vi "Format Control Table.vi"(5 "Msg Chain in":string, 7 "Controls Opt":T4, 8 "error in (no error)":errorcluster {"code" format="Error %.0f"}, 10 "Controls":T1[](array[typedef]), 11 "VIDoc Printer - Confluence In":refnum<class "VIDoc Printer - Confluence.lvclass">) -> (0 "error out":errorcluster {"code" format="Error %.0f"}, 2 "Table":string, 3 "VIDoc Printer - Confluence Out":refnum<class "VIDoc Printer - Confluence.lvclass">)   [LabVIEW 2023, in "VIDoc Printer - Confluence.lvlib" / "VIDoc Printer - Confluence.lvclass"]
uses:
  VIDoc Printer - Confluence.lvclass
  C:/projects/DMC/GitHub/DMC CLI VIDoc/Source/Documentation Generation/Printers/Printer/VIDoc Printer.lvclass
  Settings/Printer Settings/Detail Level Enum.ctl
  Parsing/TypeDefs/Controls Info Cluster.ctl
  <vilib>/picture/picture.llb/imagedata.ctl
  <vilib>/Utility/miscctls.llb/LVKeyTypeDef.ctl
  VIDoc Printer - Confluence.lvclass/VIDoc Printer - Confluence.ctl
  Accessors/Get Control Column Ordering - Full.vi
  Accessors/Get Control Column Ordering - Minimal.vi
  Accessors/Get Control Column Ordering - Standard.vi
  Accessors/Get Sortable Tables.vi
  Confluence Formatting/Confluence Formatting.lvlib
  Printer/VIDoc Printer.lvclass
  UI Interaction/UI Interaction.lvclass
  Parsing/VIDoc Parsing.lvlib
  Settings/Printer Settings/Printer Settings.lvclass
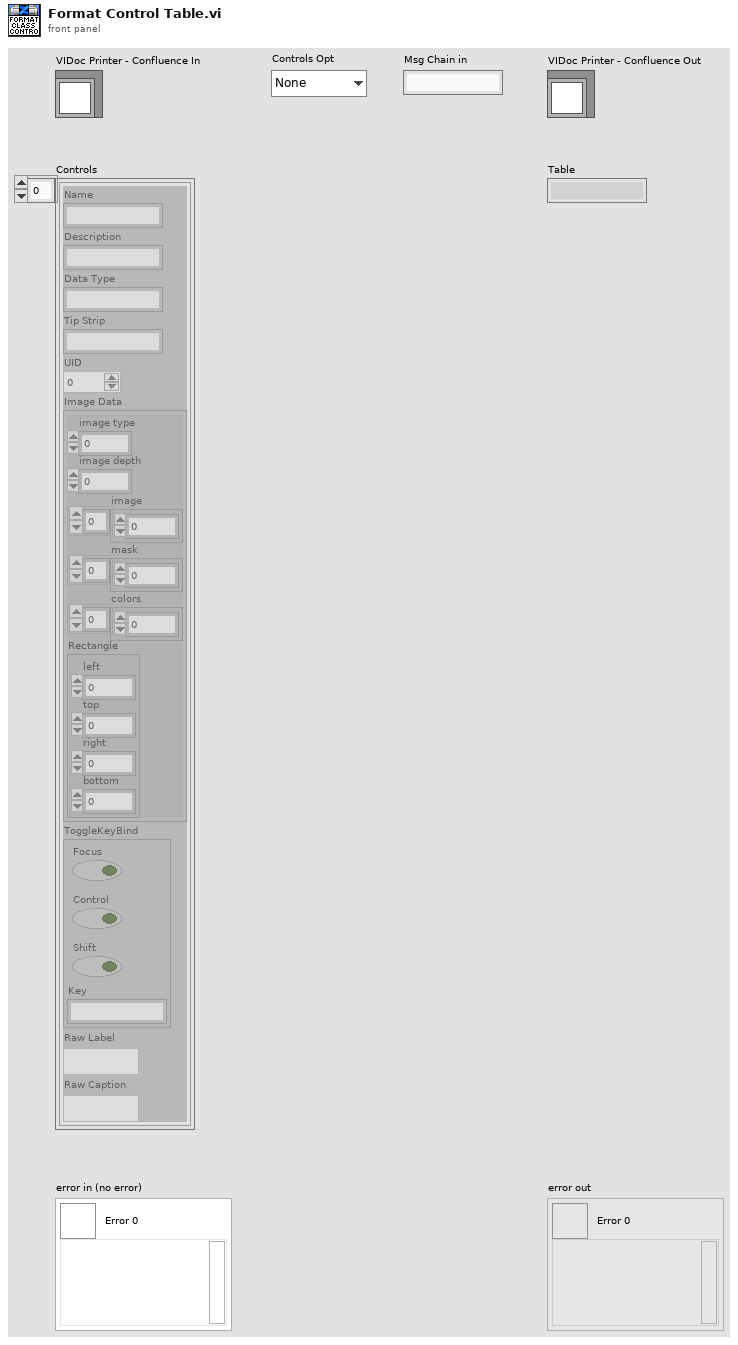
[diagram p1: front panel]
types:
  T1 = typedef "VIDoc Parsing.lvlib/Controls Info Cluster.ctl" = cluster{"Name":string, "Description":string, "Data Type":string, "Tip Strip":string, "UID":i32, "Image Data":T2, "ToggleKeyBind":T3, "Raw Label":string, "Raw Caption":string}
  T2 = typedef "imagedata.ctl" = cluster{"image type":i32, "image depth":i32, "image":u8[], "mask":u8[], "colors":u32[], "Rectangle":cluster{"left":i16, "top":i16, "right":i16, "bottom":i16}}
  T3 = typedef "LVKeyTypeDef.ctl" = cluster{"Focus":bool, "Control":bool, "Shift":bool, "Key":string}
  T4 = typedef "VIDoc Printer.lvlib/Printer Settings.lvclass/Detail Level Enum.ctl" = enum16{"None", "Minimal", "Standard", "Full"}
  T5 = typedef "VIDoc Printer - Confluence.lvlib/VIDoc Settings - Confluence.lvclass/Control Info Column.ctl" = enum16{"Image", "Name", "Description", "Caption", "Tip Strip", "Data Type", "Key Toggle"}
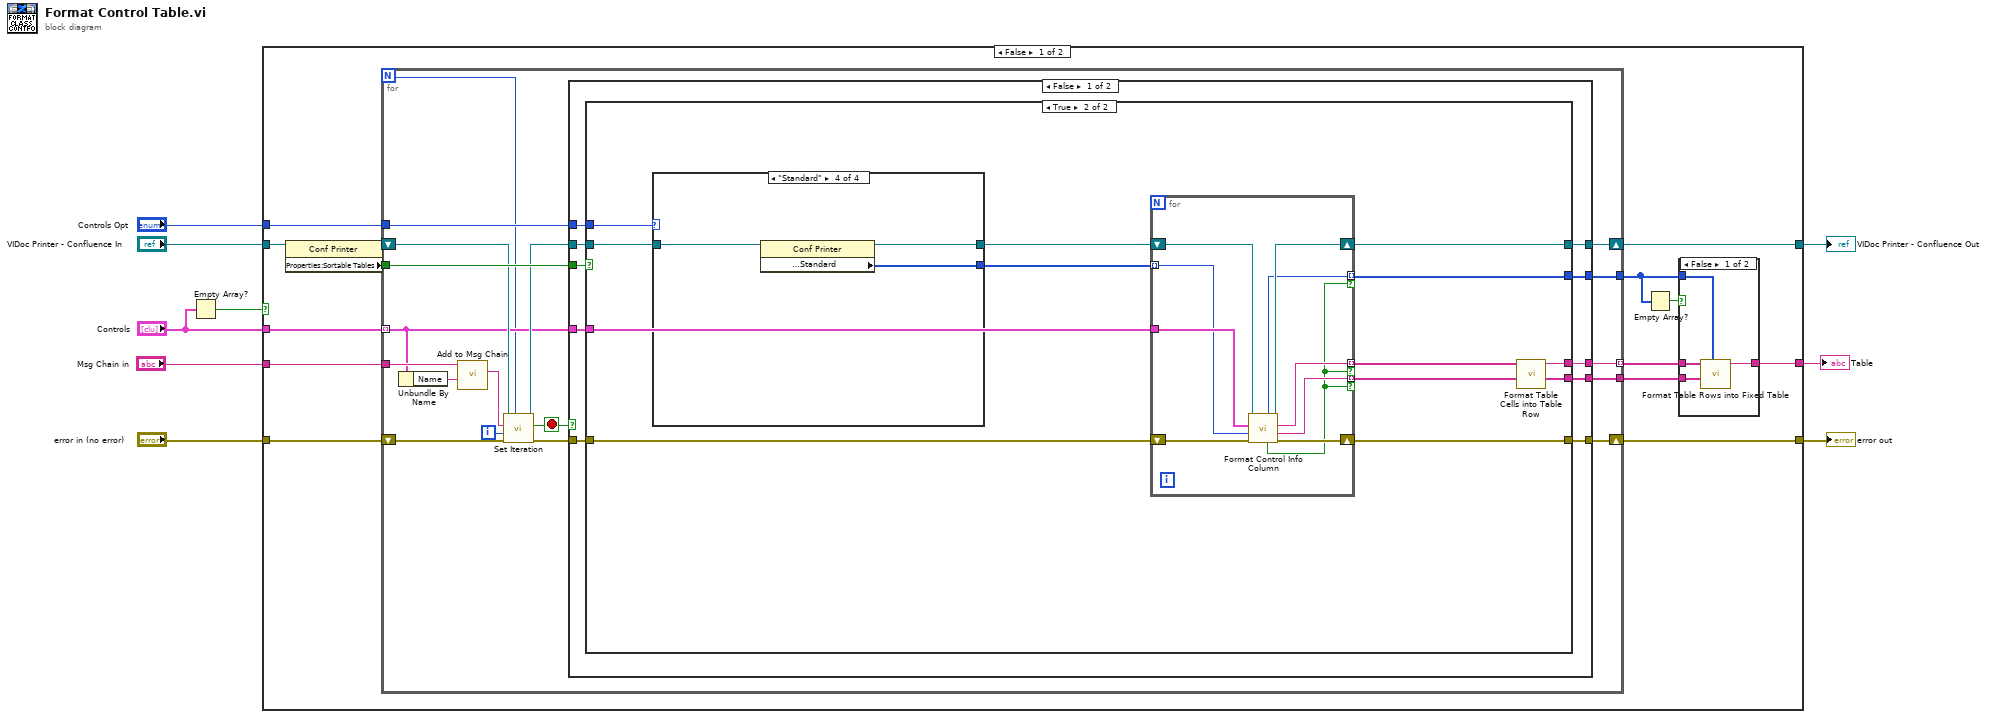
[diagram p0: block diagram]
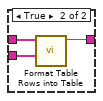
[diagram p2: hidden frame]
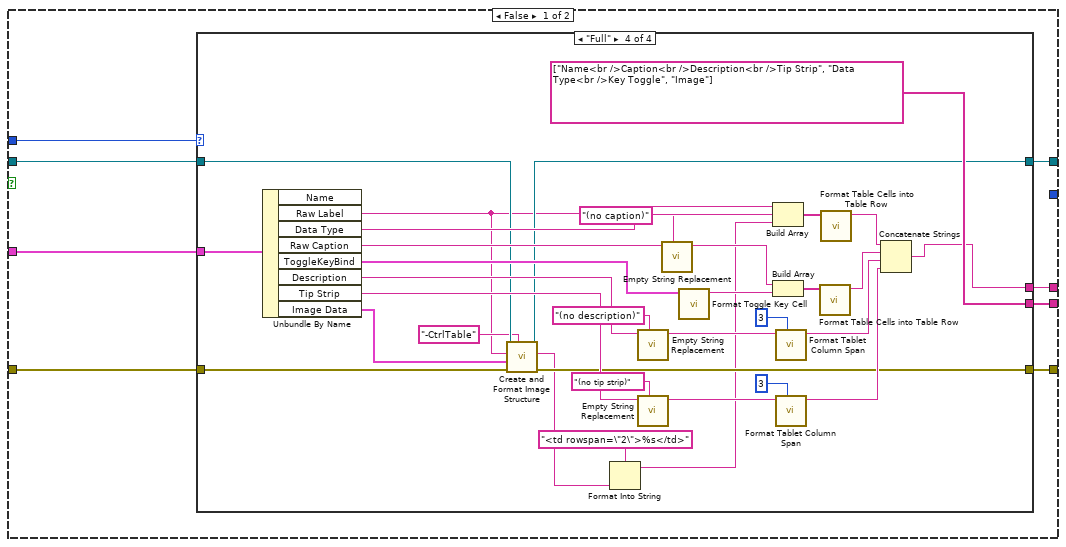
[diagram p3: hidden frame]
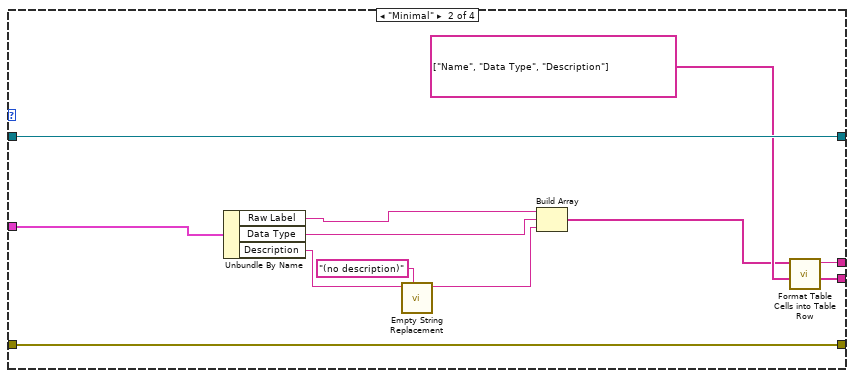
[diagram p5: hidden frame]
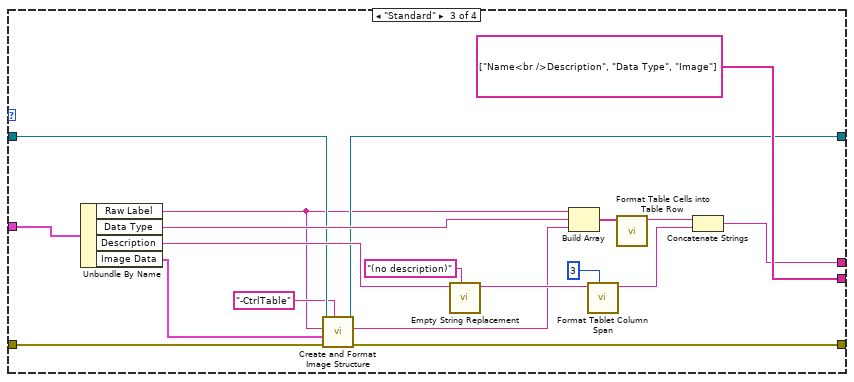
[diagram p6: hidden frame]
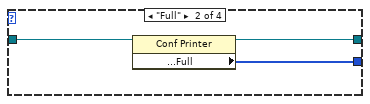
[diagram p8: hidden frame]
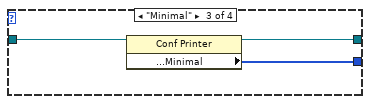
[diagram p9: hidden frame]
diagram:
  n1 = Empty Array?(array="Controls") -> (empty?=w3:bool)
  n2 = case shown="False" w3 {
    tunnel: "Controls Opt" -> [w23 _]
    tunnel: [w22 w166] -> w8
    tunnel: "error in (no error)" -> [w17 w166]
    tunnel: [w21 w167] -> w6
    tunnel: "VIDoc Printer - Confluence In" -> [w20 w167]
    tunnel: [w13 _] -> w4
    tunnel: "Controls" -> [w19 _]
    tunnel: "Msg Chain in" -> [w15 _]
    frame False {
      n3 = property class="Conf Printer"(reference=w20) -> (reference out=w16:refnum<class "VIDoc Printer - Confluence.lvclass">, "Properties:Sortable Tables"=w18:bool)  [unwired: 1 in, 1 out]
      n4 = for {
        N -> [w36]
        tunnel: w23 -> [w48]
        tunnel: w19 -> [w37] mode=indexing
        tunnel: w18 -> [w45]
        tunnel: w15 -> [w38]
        shift-right: [w47] -> w22
        shift-left: w17 -> [w42]
        shift-right: [w46] -> w21
        shift-left: w16 -> [w40]
        tunnel: [w33] -> w12 mode=indexing
        tunnel: [w32] -> w11
        tunnel: [w31] -> w10
        i -> [w35]
        stop <- w34 stop-if-true
        n5 = Unbundle By Name(w37) -> ("Name"=w44:string)
        n6 = call "Add to Msg Chain.vi"("New"=w44, "Msg Chain in"=w38) -> ("Msg Chain out"=w43:string)  [unwired: 9 in]
        n7 = call "Set Iteration.vi"("Progress Max"=w36, "error in (no error)"=w42, "Progress Value"=w35, "Message (No Message Update)"=w43, "VIDoc Printer In"=w40) -> ("error out"=w41:errorcluster, "Abort?"=w34:bool, "VIDoc Printer Out"=w39:refnum<class "VIDoc Printer - Confluence.lvclass">)  [unwired: 4 in]
        n8 = case shown="False" w34 {
          tunnel: w48 -> [w58 _]
          tunnel: [w57 w164] -> w47
          tunnel: [w56 w165] -> w46
          tunnel: w45 -> [w55 _]
          tunnel: w41 -> [w54 w164]
          tunnel: w39 -> [w53 w165]
          tunnel: w37 -> [w52 _]
          tunnel: [w51 _] -> w33
          tunnel: [w50 _] -> w32
          tunnel: [w49 _] -> w31
          frame False {
            n9 = case shown="True" w55 {
              tunnel: w58 -> [w66 w135]
              tunnel: [w65 w141] -> w57
              tunnel: [w64 w140] -> w56
              tunnel: w54 -> [w63 w142]
              tunnel: w53 -> [w62 w132]
              tunnel: w52 -> [w61 w139]
              tunnel: [w60 w143] -> w51
              tunnel: [w59 w136] -> w50
              tunnel: [_ w138] -> w49
              frame False {
                n10 = case shown="\"Full\"" w66 {
                  tunnel: [w68 w77 w86 w106] -> w65
                  tunnel: w63 -> [w68 w77 w87 w107]
                  tunnel: [w67 w79 w84 w104] -> w64
                  tunnel: w62 -> [w67 w79 w85 w105]
                  tunnel: w61 -> [_ w78 w98 w131]
                  tunnel: [_ w74 w90 w115] -> w60
                  tunnel: [_ string[] ["Name", "Data Type", "Description"] ("Table Headers") string[] ["Name<br />Description", "Data Type", "Image"] ("Table Headers") string[] ["Name<br />Caption<br />Description<br />Tip Strip", "Data Type<br />Key Toggle", "Image"] ("Table Headers")] -> w59
                  frame "None" {
                  }
                  frame "Minimal" {
                    n11 = Unbundle By Name(w78) -> ("Raw Label"=w69:string, "Data Type"=w73:string, "Description"=w72:string)
                    n12 = call "Empty String Replacement.vi"("Empty"="(no description)", "String"=w72) -> ("String Out"=w70:string)  [unwired: 9 in]
                    n13 = Build Array(w69, w73, w70) -> (w75:string[])
                    n14 = call "Format Table Cells into Table Row.vi"("Table Cells"=w75) -> ("Table Row Text"=w74:string)  [unwired: 10 in]
                  }
                  frame "Standard" {
                    n15 = Unbundle By Name(w98) -> ("Raw Label"=w82:string, "Data Type"=w96:string, "Description"=w95:string, "Image Data"=w81:T2)
                    n16 = call "Create and Format Image Structure.vi"("Name Addition"="-CtrlTable" ("string"), "Error in"=w87, "Image Data"=w81, "Name"=w82, "VIDoc Printer - Confluence In"=w85) -> ("Error out"=w86:errorcluster, "Image Structure Text"=w80:string, "VIDoc Printer - Confluence Out"=w84:refnum<class "VIDoc Printer - Confluence.lvclass">)  [unwired: 3 in, 1 out]
                    n17 = call "Empty String Replacement.vi"("Empty"="(no description)", "String"=w95) -> ("String Out"=w93:string)  [unwired: 9 in]
                    n18 = Build Array(w82, w96, w80) -> (w89:string[])
                    n19 = call "Format Tablet Column Span.vi"("Column Count"=3, "Spanned Cell Text"=w93) -> ("Row Text"=w91:string)  [unwired: 9 in]
                    n20 = call "Format Table Cells into Table Row.vi"("Table Cells"=w89) -> ("Table Row Text"=w88:string)  [unwired: 10 in]
                    n21 = Concatenate Strings(w88, w91) -> (w90:string)
                  }
                  frame "Full" {
                    n22 = Unbundle By Name(w131) -> ("Raw Label"=w102:string, "Data Type"=w129:string, "Raw Caption"=w118:string, "ToggleKeyBind"=w117:T3, "Description"=w128:string, "Tip Strip"=w119:string, "Image Data"=w101:T2)  [unwired: 1 out]
                    n23 = call "Create and Format Image Structure.vi"("Name Addition"="-CtrlTable" ("string"), "Error in"=w107, "Image Data"=w101, "Name"=w102, "VIDoc Printer - Confluence In"=w105) -> ("Error out"=w106:errorcluster, "Image Structure Text"=w100:string, "VIDoc Printer - Confluence Out"=w104:refnum<class "VIDoc Printer - Confluence.lvclass">)  [unwired: 3 in, 1 out]
                    n24 = Format Into String(format string="<td rowspan=\"2\">%s</td>", w100) -> (resulting string=w99:string)  [unwired: 2 in, 1 out]
                    n25 = call "Empty String Replacement.vi"("Empty"="(no description)", "String"=w128) -> ("String Out"=w126:string)  [unwired: 9 in]
                    n26 = call "Empty String Replacement.vi"("Empty"="(no tip strip)", "String"=w119) -> ("String Out"=w121:string)  [unwired: 9 in]
                    n27 = call "Empty String Replacement.vi"("Empty"="(no caption)", "String"=w118) -> ("String Out"=w110:string)  [unwired: 9 in]
                    n28 = call "Format Toggle Key Cell.vi"("ToggleKeyBind"=w117) -> ("Toggle Key Text"=w116:string)  [unwired: 9 in, 1 out]
                    n29 = Build Array(w102, w129, w99) -> (w114:string[])
                    n30 = Build Array(w110, w116) -> (w112:string[])
                    n31 = call "Format Tablet Column Span.vi"("Column Count"=3, "Spanned Cell Text"=w126) -> ("Row Text"=w124:string)  [unwired: 9 in]
                    n32 = call "Format Tablet Column Span.vi"("Column Count"=3, "Spanned Cell Text"=w121) -> ("Row Text"=w120:string)  [unwired: 9 in]
                    n33 = call "Format Table Cells into Table Row.vi"("Table Cells"=w112) -> ("Table Row Text"=w111:string)  [unwired: 10 in]
                    n34 = call "Format Table Cells into Table Row.vi"("Table Cells"=w114) -> ("Table Row Text"=w113:string)  [unwired: 10 in]
                    n35 = Concatenate Strings(w113, w111, w124, w120) -> (w115:string)
                  }
                }
              }
              frame True {
                n36 = case shown="\"Standard\"" w135 {
                  tunnel: [_ w145 w148 w151] -> w134
                  tunnel: [w144 w146 w149 w152] -> w133
                  tunnel: w132 -> [w144 w147 w150 w153]
                  frame "None" {
                  }
                  frame "Full" {
                    n37 = property class="Conf Printer"(reference=w147) -> (reference out=w146:refnum<class "VIDoc Printer - Confluence.lvclass">, "Properties:Table Column Ordering:Control:Full"=w145:T5[])  [unwired: 1 in, 1 out]
                  }
                  frame "Minimal" {
                    n38 = property class="Conf Printer"(reference=w150) -> (reference out=w149:refnum<class "VIDoc Printer - Confluence.lvclass">, "Properties:Table Column Ordering:Control:Minimal"=w148:T5[])  [unwired: 1 in, 1 out]
                  }
                  frame "Standard" {
                    n39 = property class="Conf Printer"(reference=w153) -> (reference out=w152:refnum<class "VIDoc Printer - Confluence.lvclass">, "Properties:Table Column Ordering:Control:Standard"=w151:T5[])  [unwired: 1 in, 1 out]
                  }
                }
                n40 = for {
                  tunnel: w139 -> [w159]
                  shift-right: [w162] -> w141
                  shift-left: w142 -> [w163]
                  shift-right: [w160] -> w140
                  shift-left: w133 -> [w161]
                  tunnel: [w158] -> w138 mode=indexing if=w155
                  tunnel: [w157] -> w137 mode=indexing if=w155
                  tunnel: [w156] -> w136 mode=indexing if=w155
                  tunnel: w134 -> [w154] mode=indexing
                  n41 = call "Format Control Info Column.vi"("error in (no error)"=w163, "Column"=w154, "Control Info Cluster"=w159, "VIDoc Printer - Confluence In"=w161) -> ("error out"=w162:errorcluster, "Header"=w156:string, "Cell Text"=w157:string, "VIDoc Printer - Confluence Out"=w160:refnum<class "VIDoc Printer - Confluence.lvclass">, "Viable Value?"=w155:bool, "Pixel Width"=w158:i16)  [unwired: 2 in]
                }
                n42 = call "Format Table Cells into Table Row.vi"("Table Cells"=w137) -> ("Table Row Text"=w143:string)  [unwired: 10 in]
              }
            }
          }
          frame True {
          }
        }
      }
      n43 = Empty Array?(array=w10) -> (empty?=w14:bool)
      n44 = case shown="False" w14 {
        tunnel: w12 -> [w26 w30]
        tunnel: [w24 w29] -> w13
        tunnel: w11 -> [w27 w28]
        tunnel: w10 -> [w25 _]
        frame False {
          n45 = call "Format Table Rows into Fixed Table.vi"("Column Pixel Widths"=w25, "Table Headers"=w27, "Table Rows"=w26) -> ("Table Text"=w24:string)  [unwired: 8 in]
        }
        frame True {
          n46 = call "Format Table Rows into Table.vi"("Table Headers"=w28, "Table Rows"=w30) -> ("Table Text"=w29:string)  [unwired: 9 in]
        }
      }
    }
    frame True {
    }
  }
  "error out" <- w8
  "VIDoc Printer - Confluence Out" <- w6
  "Table" <- w4
